vi "Test Alt Window.vi"() -> ()   [LabVIEW 2013]
uses:
  <vilib>/Platform/TimedLoop/XDataNode/timing_clust.ctl
  <vilib>/Platform/TimedLoop/XDataNode/nitl_modes.ctl
  <vilib>/Platform/TimedLoop/XDataNode/wakeup.ctl
  <vilib>/Platform/TimedLoop/XDataNode/XDataNode.xnode
  <vilib>/Platform/TimedLoop/XDataNode/XDNodeRunTimeDep.lvlib
panel:
  in  "Stop":bool
  in  "Msg":string
  in  "Altitude":dbl format="%#_13g"
  in  "Visible":bool
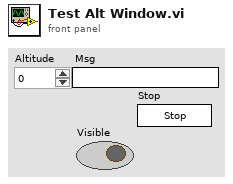
[diagram p1: front panel]
types:
  T1 = cluster{"Heading":string, "Altitude":dbl, "Visible?":bool}
  T2 = typedef "XDNodeRunTimeDep.lvlib/timing_clust.ctl" = cluster{"Expected End [f-1]":u64, "Actual End [f-1]":u64, "Finished Late? [f-1]":bool, "Expected End [i-1]":u64, "Actual End [i-1]":u64, "Finished Late? [i-1]":bool, "Expected Start [i]":u64, "Actual Start [i]":u64, "Expected Start [f]":u64, "Actual Start [f]":u64, "Source Name":string, "Structure Name":string, "Period":i64, "Deadline":i64, "Offset":i64, "Start":i64, "Priority":i32, "Timeout":i32, "Mode":T3, "Wakeup Reason":T4, "Error":errorcluster, "Source Type":string, "Secondary Source Type":string, "Global End Time":u64, "Global Start Time":u64, "Frame Duration":u64, "Iteration Duration":u64, "Assigned CPU":i32, "I/O Scan Engine Mode":u32}
  T3 = typedef "XDNodeRunTimeDep.lvlib/nitl_modes.ctl" = enum32{"No Change", "Process missed periods, maintain original phase", "Discard missed periods, maintain original phase", "Process missed periods, ignore original phase", "Discard missed periods, ignore original phase"}
  T4 = typedef "XDNodeRunTimeDep.lvlib/wakeup.ctl" = enum32{"Normal", "Aborted", "Asynchronous wakeup", "Timing source error", "Timed loop error", "Timeout"}
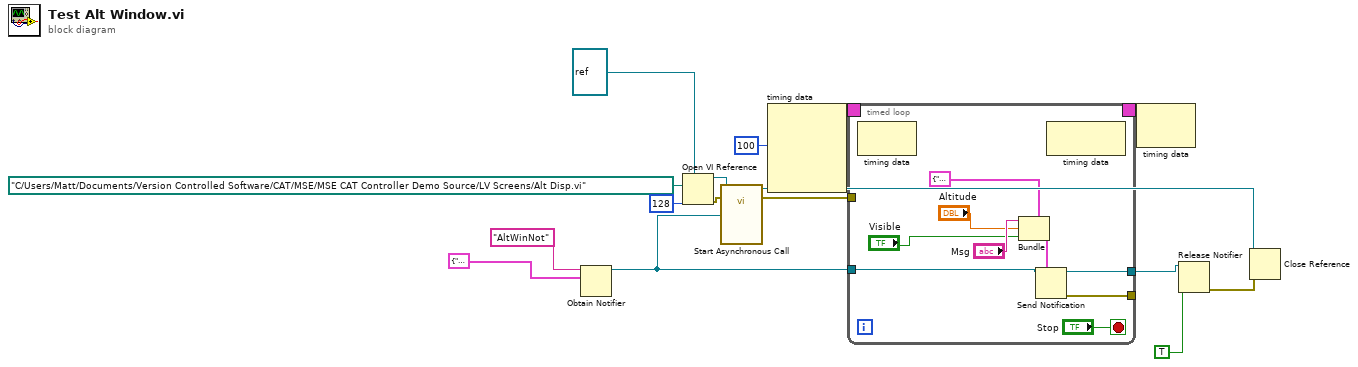
[diagram p0: block diagram]
diagram:
  n1 = Obtain Notifier(name (unnamed)="AltWinNot", notification data type=T1 {"Heading"="Current Effective Altitude in  Feet", "Altitude"=0.0, "Visible?"=TRUE}) -> (notifier out=w2:refnum<notifier>)  [unwired: 2 in, 2 out]
  n2 = Open VI Reference(type specifier VI Refnum (for type only)=refnum<vi> refnum, vi path=path "C:/Users/Matt/Documents/Version Controlled Software/CAT/MSE/MSE CAT Controller Demo Source/LV Screens/Alt Disp.vi", options=128) -> (vi reference=w14:refnum<vi>, error out=w13:errorcluster)  [unwired: 3 in]
  n3 = call-by-ref "Start Asynchronous Call"(reference=w14, error in=w13, "Notifer In"=w2) -> (reference out=w3:refnum<vi>, error out=w4:errorcluster)  [unwired: 3 in]
  n4 = node-c288(i64 100 ("Period")) -> (w10:T2)  [unwired: 3 in]
  n5 = timed-loop {
    tunnel: w2 -> [w20]
    timing: w10 -> [_]
    timing-out: [_] -> w9
    tunnel: [w19] -> w7
    tunnel: w4 -> [_]
    tunnel: [w17] -> _
    stop <- "Stop" stop-if-true
    n6 = node-c288() -> ()  [unwired: 1 in, 1 out]
    n7 = Bundle(cluster=T1 {"Heading"="Current Effective Altitude in  Feet", "Altitude"=0.0, "Visible?"=TRUE}, "Heading"="Msg", "Altitude"="Altitude", "Visible?"="Visible") -> (w21:T1)
    n8 = Send Notification(notification=w21, notifier=w20) -> (notifier out=w19:refnum<notifier>, error out=w17:errorcluster)  [unwired: 1 in]
    n9 = node-c288() -> ()  [unwired: 1 in, 1 out]
  }
  n10 = node-c288(w9) -> ()  [unwired: 1 out]
  n11 = Release Notifier(notifier=w7, force destroy? (F)=TRUE) -> (error out=w6:errorcluster)  [unwired: 1 in, 2 out]
  n12 = Close Reference(reference=w3, error in (no error)=w6) -> ()  [unwired: 1 out]
